vi "DeRemapResource.vi"(4 "prb_num":dbl, 5 "error in (no error)":errorcluster caption="错误输入（无错误）", 7 "Nu":dbl, 8 "Nsym_slot":dbl, 9 "defredata":cdb[](array[numeric]), 10 "appended path":path) -> (0 "error IO":errorcluster, 1 "deremapdata":cdb[][](array[numeric]))   [LabVIEW 2015]
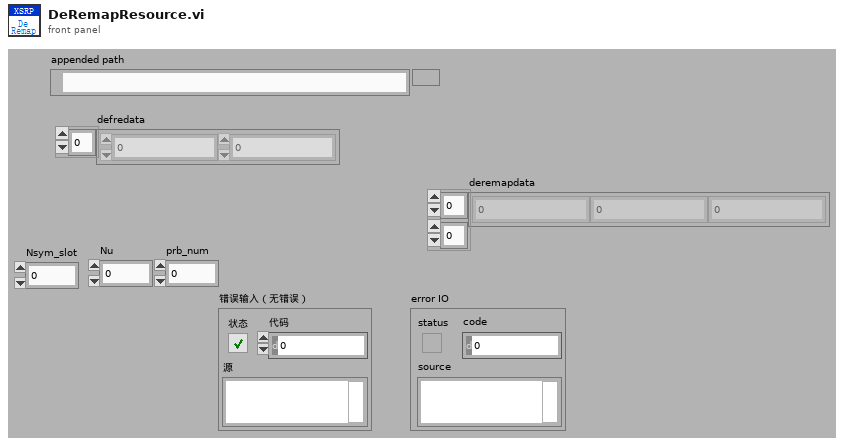
[diagram p1: front panel]
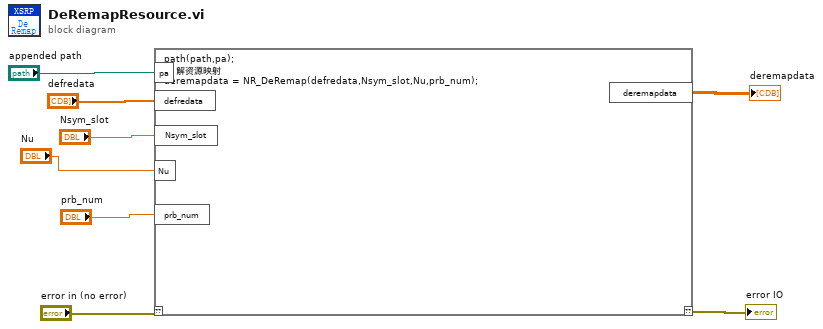
[diagram p0: block diagram]
diagram:
  n1 = script code="path(path,pa);\n% 解资源映射\nderemapdata = NR_DeRemap(defredata,Nsym_slot,Nu,prb_num);"("??"="error in (no error)", "pa"="appended path", "defredata"="defredata", "Nsym_slot"="Nsym_slot", "Nu"="Nu", "prb_num"="prb_num") -> ("??"=→"error IO":errorcluster, "deremapdata"=→"deremapdata":cdb[][])
